vi "Read Item Path.vi"(8 "error in (no error)":errorcluster, 11 "LabVIEWItem in":refnum<class "LabVIEWItem.lvclass">) -> (0 "error out":errorcluster, 2 "Item Path":path, 3 "LabVIEWItem out":refnum<class "LabVIEWItem.lvclass">)   [LabVIEW 2019, in "Panther Dashboard.lvlib" / "LabVIEWItem.lvclass"]
uses:
  LabVIEWItem.lvclass
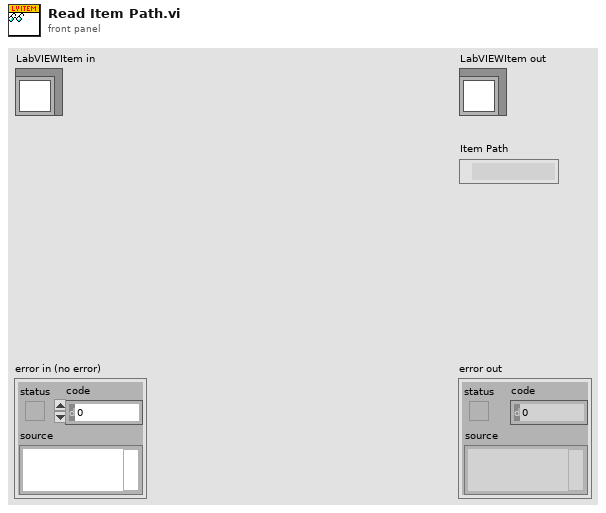
[diagram p1: front panel]
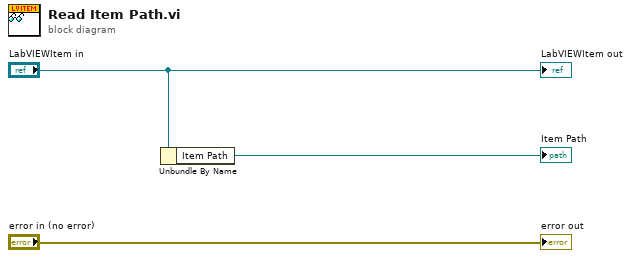
[diagram p0: block diagram]
diagram:
  n1 = Unbundle By Name("LabVIEWItem in") -> ("Item Path"=→"Item Path":path)
  "error out" <- "error in (no error)"
  "LabVIEWItem out" <- "LabVIEWItem in"
